vi "set_Sim_Alg_Class.vi"(8 "error in (no error)":errorcluster, 10 "SimAlg.lvclass":refnum<class "PrllPerElmnt.lvclass">, 11 "QuWire in":refnum<class "QuWire.lvclass">) -> (0 "error out":errorcluster, 3 "QuWire out":refnum<class "QuWire.lvclass">)   [LabVIEW 2020, in "QuWire.lvclass"]
uses:
  QuWire.lvclass
  SimAlg/PrllPerElement/PrllPerElmnt.lvclass
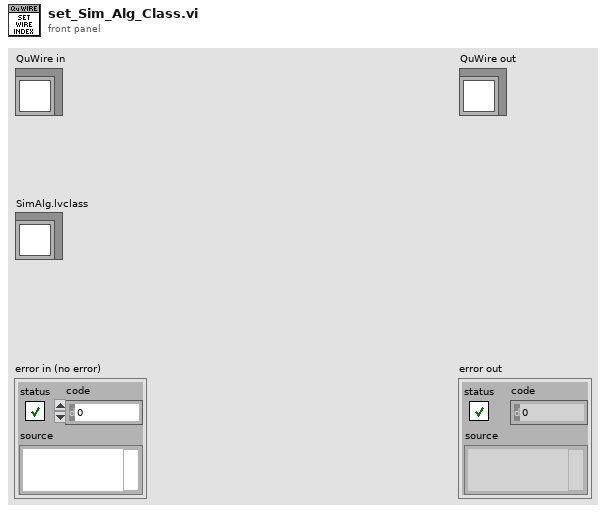
[diagram p1: front panel]
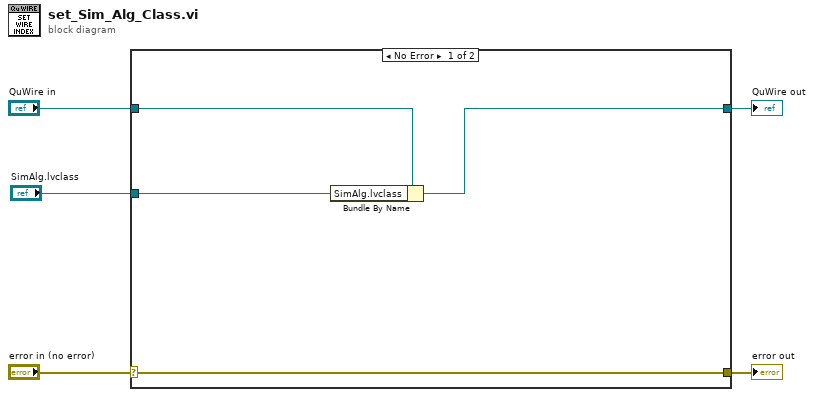
[diagram p0: block diagram]
diagram:
  n1 = case shown="No Error" "error in (no error)" {
    selector: "error in (no error)" -> [w9 w11]
    tunnel: [w9 w11] -> w4
    tunnel: [w7 w10] -> w2
    tunnel: "QuWire in" -> [w8 w10]
    tunnel: "SimAlg.lvclass" -> [w6 _]
    frame No Error {
      n2 = Bundle By Name(cluster=w8, "SimAlg.lvclass"=w6) -> (w7:refnum<class "QuWire.lvclass">)
    }
    frame Error {
    }
  }
  "error out" <- w4
  "QuWire out" <- w2
